vi "Test Check Packets.vi"() -> ()   [LabVIEW 2022 SP3, in "AoC22.lvlib"]
uses:
  AoC22.lvlib
panel:
  out "Correct Order?":bool
  in  "Pair":string="[[4,4],4,4]\n[[4,4],4,4,4]"
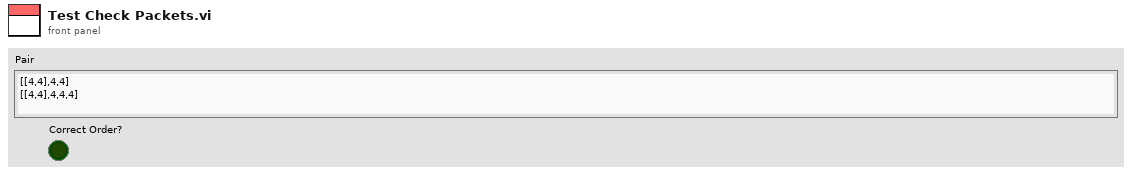
[diagram p1: front panel]
types:
  T1 = typedef "AoC22.lvlib/Packet Item.ctl" = cluster{"Depth":i32, "Value":i32}
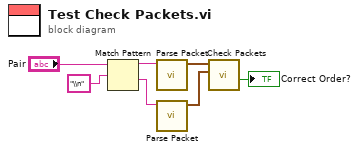
[diagram p0: block diagram]
diagram:
  n1 = Match Pattern(string="Pair", regular expression="\\n") -> (before substring=w3:string, after substring=w2:string)  [unwired: 1 in, 2 out]
  n2 = call "Parse Packet.vi"("Packet"=w3) -> ("Packet Data"=w5:T1[])  [unwired: 10 in]
  n3 = call "Parse Packet.vi"("Packet"=w2) -> ("Packet Data"=w4:T1[])  [unwired: 10 in]
  n4 = call "Check Packets.vi"("Right"=w4, "Left"=w5) -> ("Correct Order?"=→"Correct Order?":bool)  [unwired: 9 in]
